vi "Read Hardware Interface Configuration.vi"(8 "error in (no error)":errorcluster, 10 "hardware interface index":u16, 11 "PLBB in":refnum<class "PL BlackBox Modbus Client.lvclass">) -> (0 "error out":errorcluster, 2 "hardware interface configuration":T1 {"UART"."flow control" items=["none", "rts", "cts", "rts/cts"]; "UART"."stop bits" items=["1", "1.5", "2"]; "UART"."parity" items=["none", "even", "odd"]}, 3 "PLBB out":refnum<class "PL BlackBox Modbus Client.lvclass">)   [LabVIEW 2015, in "PL BlackBox Modbus Client.lvclass"]
doc: "Reads the hardware interface configuration."
uses:
  PL BlackBox Modbus Client.lvclass
  <vilib>/plasmapper/PL Modbus Client/PL Modbus Client.lvclass
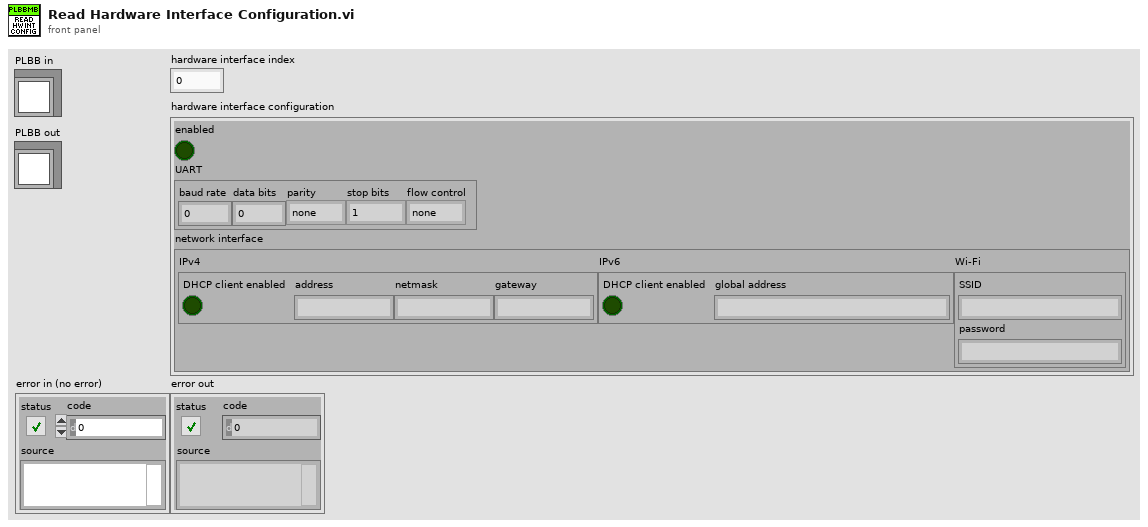
[diagram p1: front panel]
types:
  T1 = cluster{"enabled":bool, "UART":cluster{"baud rate":u32, "data bits":u16, "parity":u16, "stop bits":u16, "flow control":u16}, "network interface":cluster{"IPv4":cluster{"DHCP client enabled":bool, "address":string, "netmask":string, "gateway":string}, "IPv6":cluster{"DHCP client enabled":bool, "global address":string}, "Wi-Fi":cluster{"SSID":string, "password":string}}}
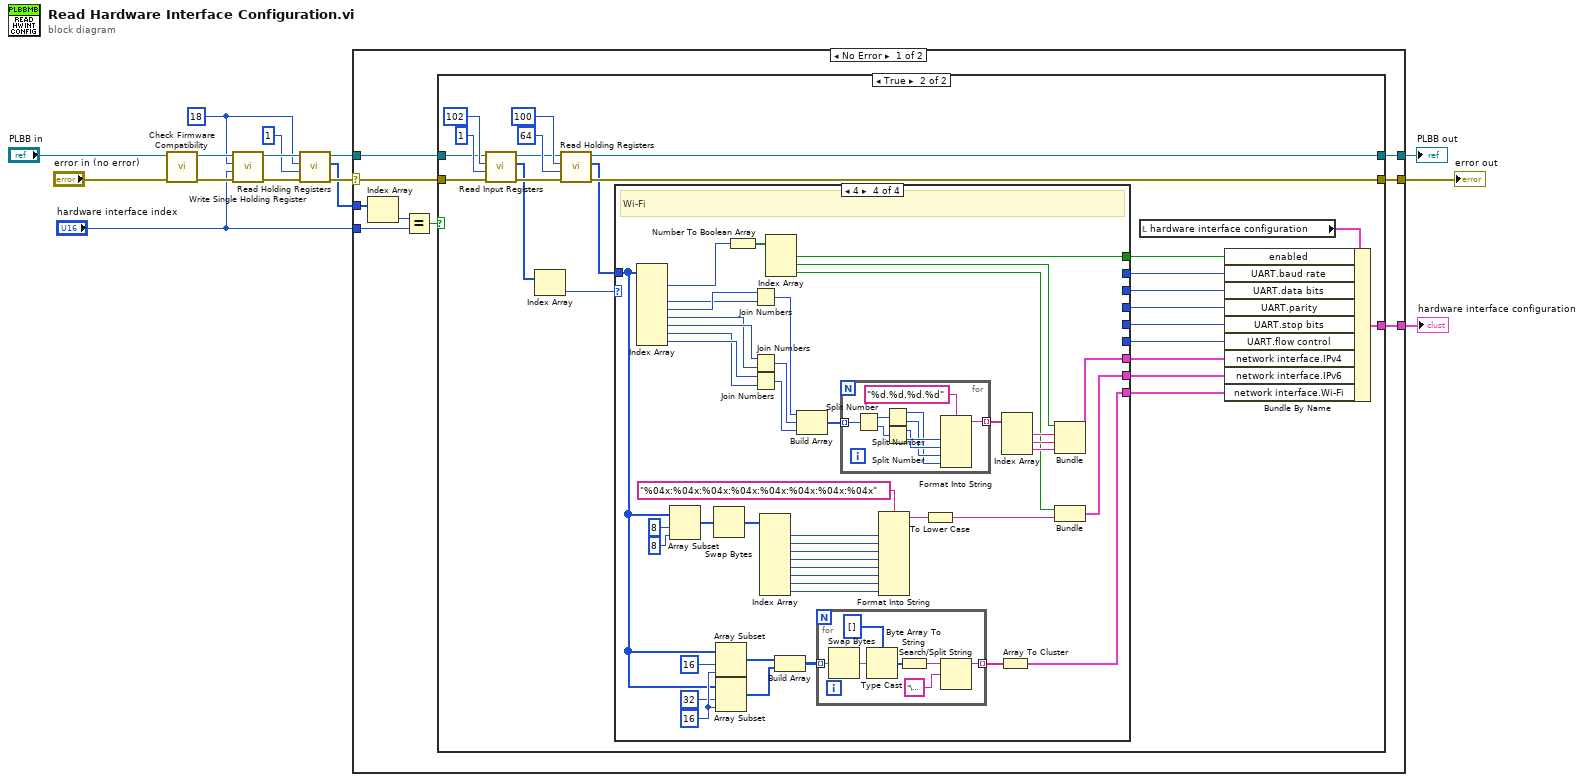
[diagram p0: block diagram]
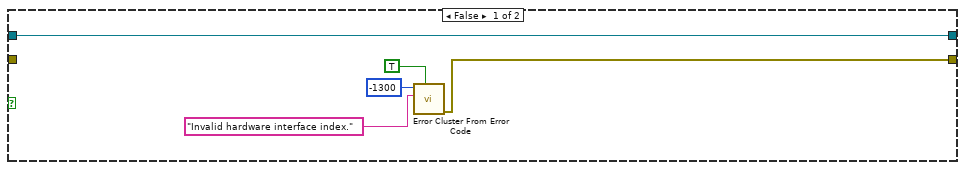
[diagram p2: hidden frame]
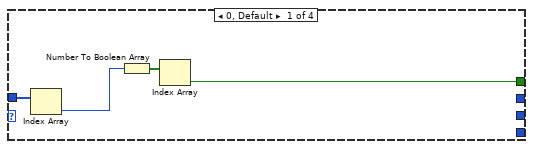
[diagram p3: hidden frame]
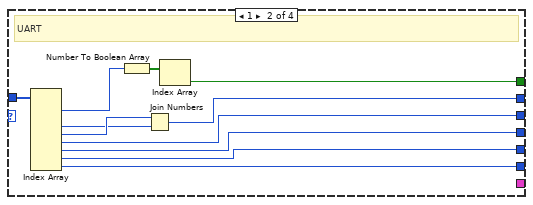
[diagram p4: hidden frame]
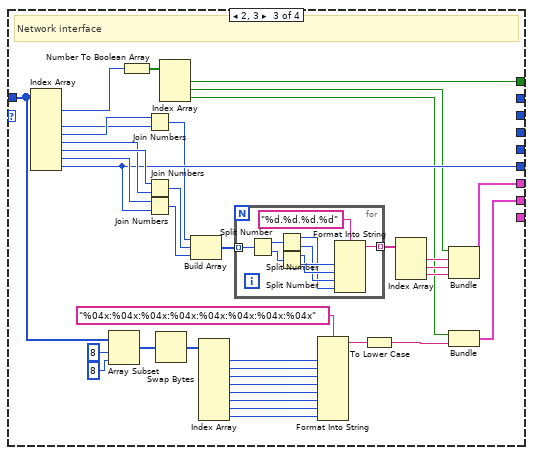
[diagram p5: hidden frame]
diagram:
  w7 = u16 18 ("address")
  n1 = call-dynamic "Check Firmware Compatibility.vi"("error in (no error)"="error in (no error)", "PLBB in"="PLBB in") -> ("error out"=w10:errorcluster, "PLBB out"=w11:refnum<class "PL BlackBox Modbus Client.lvclass">)  [unwired: 8 in]
  n2 = call <vilib>:"Write Single Holding Register.vi"("error in (no error)"=w10, "value"="hardware interface index", "address"=w7, "MODBUS in"=w11) -> ("error out"=w6:errorcluster, "MODBUS out"=w9:refnum<class "PL BlackBox Modbus Client.lvclass">)  [unwired: 6 in]
  n3 = call <vilib>:"Read Holding Registers.vi"("error in (no error)"=w6, "number of holding registers"=u16 1 ("address"), "address"=w7, "MODBUS in"=w9) -> ("error out"=w5:errorcluster, "values"=w3:u16[], "MODBUS out"=w4:refnum<class "PL BlackBox Modbus Client.lvclass">)  [unwired: 5 in]
  n4 = case shown="No Error" w5 {
    selector: w5 -> [w17 w176]
    tunnel: [w24 w176] -> w15
    tunnel: [w23 w177] -> w14
    tunnel: w4 -> [w18 w177]
    tunnel: w3 -> [w22 _]
    tunnel: "hardware interface index" -> [w20 _]
    tunnel: [w16 _] -> w1
    frame No Error {
      n5 = Index Array(array=w22) -> (element=w21:u16)  [unwired: 1 in]
      n6 = Equal?(x=w21, y=w20) -> (x = y?=w19:bool)
      n7 = case shown="True" w19 {
        tunnel: [w25 w53] -> w24
        tunnel: [w29 w52] -> w23
        tunnel: w18 -> [w29 w38]
        tunnel: w17 -> [_ w37]
        tunnel: [_ w48] -> w16
        frame False {
          n8 = call <vilib>:"Error Cluster From Error Code.vi"("show call chain? (False)"=TRUE, "error message (\"\")"="Invalid hardware interface index." ("error message (\"\")"), "error code (0)"=-1300) -> ("error out"=w25:errorcluster)  [unwired: 6 in]
        }
        frame True {
          n9 = call <vilib>:"Read Input Registers.vi"("error in (no error)"=w37, "number of input registers"=u16 1 ("address"), "address"=u16 102, "MODBUS in"=w38) -> ("error out"=w36:errorcluster, "values"=w34:u16[], "MODBUS out"=w35:refnum<class "PL BlackBox Modbus Client.lvclass">)  [unwired: 5 in]
          n10 = Index Array(array=w34) -> (element=w33:u16)  [unwired: 1 in]
          n11 = call <vilib>:"Read Holding Registers.vi"("error in (no error)"=w36, "number of holding registers"=u16 64 ("address"), "address"=u16 100, "MODBUS in"=w35) -> ("error out"=w53:errorcluster, "values"=w41:u16[], "MODBUS out"=w52:refnum<class "PL BlackBox Modbus Client.lvclass">)  [unwired: 5 in]
          n12 = case shown="4" w33 {
            tunnel: [w55 w66 w103 w157] -> w47
            tunnel: [_ w63 _ _] -> w46
            tunnel: [_ w62 _ _] -> w45
            tunnel: [_ w61 _ _] -> w44
            tunnel: [_ w60 w97 _] -> w43
            tunnel: [_ w59 _ _] -> w42
            tunnel: w41 -> [w54 w58 w78 w129]
            tunnel: [_ _ w87 w136] -> w32
            tunnel: [_ _ w85 w133] -> w31
            tunnel: [_ _ _ w131] -> w30
            frame 0, Default {
              n13 = Index Array(array=w54) -> (element=w57:u16)  [unwired: 1 in]
              n14 = Number To Boolean Array(number=w57) -> (Boolean array=w56:bool[])
              n15 = Index Array(array=w56) -> (element=w55:bool)  [unwired: 1 in]
            }
            frame 1 {
              # "UART"
              n16 = Index Array(array=w58) -> (element #1=w68:u16, element #3=w64:u16, element #4=w65:u16, element #5=w62:u16, element #6=w63:u16, element #7=w61:u16, element #8=w60:u16)  [unwired: 8 in, 1 out]
              n17 = Number To Boolean Array(number=w68) -> (Boolean array=w67:bool[])
              n18 = Join Numbers(hi=w65, lo=w64) -> ((hi.lo)=w59:u32)
              n19 = Index Array(array=w67) -> (element=w66:bool)  [unwired: 1 in]
            }
            frame 2, 3 {
              # "Network interface"
              n20 = Index Array(array=w78) -> (element #1=w105:u16, element #3=w101:u16, element #4=w102:u16, element #5=w99:u16, element #6=w100:u16, element #7=w98:u16, element #8=w97:u16)  [unwired: 8 in, 1 out]
              n21 = Array Subset(array=w78, index=8, length=8) -> (w82:u16[])
              n22 = Number To Boolean Array(number=w105) -> (Boolean array=w104:bool[])
              n23 = Join Numbers(hi=w102, lo=w101) -> ((hi.lo)=w96:u32)
              n24 = Join Numbers(hi=w100, lo=w99) -> ((hi.lo)=w95:u32)
              n25 = Join Numbers(hi=w98, lo=w97) -> ((hi.lo)=w94:u32)
              n26 = Swap Bytes(anything=w82) -> (byte swapped=w69:u16[])
              n27 = Index Array(array=w104) -> (element #1=w103:bool, element #2=w88:bool, element #3=w86:bool)  [unwired: 3 in]
              n28 = Build Array(w96, w95, w94) -> (w93:u32[])
              n29 = Index Array(array=w69) -> (element #1=w77:u16, element #2=w76:u16, element #3=w75:u16, element #4=w74:u16, element #5=w73:u16, element #6=w72:u16, element #7=w71:u16, element #8=w70:u16)  [unwired: 8 in]
              n30 = for {
                tunnel: w93 -> [w114] mode=indexing
                tunnel: [w106] -> w92 mode=indexing
                n31 = Split Number(x=w114) -> (hi(x)=w113:u16, lo(x)=w112:u16)
                n32 = Split Number(x=w113) -> (hi(x)=w107:u8, lo(x)=w108:u8)
                n33 = Split Number(x=w112) -> (hi(x)=w109:u8, lo(x)=w110:u8)
                n34 = Format Into String(format string="%d.%d.%d.%d", w110, w109, w108, w107) -> (resulting string=w106:string)  [unwired: 2 in, 1 out]
              }
              n35 = Format Into String(format string="%04x:%04x:%04x:%04x:%04x:%04x:%04x:%04x", w77, w76, w75, w74, w73, w72, w71, w70) -> (resulting string=w83:string)  [unwired: 2 in, 1 out]
              n36 = To Lower Case(string=w83) -> (all lower case string=w79:string)
              n37 = Index Array(array=w92) -> (element #1=w91:string, element #2=w89:string, element #3=w90:string)  [unwired: 3 in]
              n38 = Bundle(w88, w91, w89, w90) -> (w87:cluster{bool, string, string, string})  [unwired: 1 in]
              n39 = Bundle(w86, w79) -> (w85:cluster{bool, string})  [unwired: 1 in]
            }
            frame 4 {
              w143 = 16 ("index")
              # "Wi-Fi"
              n40 = Index Array(array=w129) -> (element #1=w159:u16, element #3=w155:u16, element #4=w156:u16, element #5=w153:u16, element #6=w154:u16, element #7=w115:u16, element #8=w116:u16)  [unwired: 8 in, 1 out]
              n41 = Array Subset(array=w129, index=8, length=8) -> (w128:u16[])
              n42 = Swap Bytes(anything=w128) -> (byte swapped=w117:u16[])
              n43 = Array Subset(array=w129, index=16, length=w143) -> (w144:u16[])
              n44 = Array Subset(array=w129, index=32, length=w143) -> (w145:u16[])
              n45 = Number To Boolean Array(number=w159) -> (Boolean array=w158:bool[])
              n46 = Join Numbers(hi=w156, lo=w155) -> ((hi.lo)=w152:u32)
              n47 = Join Numbers(hi=w154, lo=w153) -> ((hi.lo)=w151:u32)
              n48 = Join Numbers(hi=w116, lo=w115) -> ((hi.lo)=w150:u32)
              n49 = Index Array(array=w117) -> (element #1=w125:u16, element #2=w124:u16, element #3=w123:u16, element #4=w122:u16, element #5=w121:u16, element #6=w120:u16, element #7=w119:u16, element #8=w118:u16)  [unwired: 8 in]
              n50 = Index Array(array=w158) -> (element #1=w157:bool, element #2=w137:bool, element #3=w134:bool)  [unwired: 3 in]
              n51 = Build Array(w144, w145) -> (w146:u16[][])
              n52 = Build Array(w152, w151, w150) -> (w149:u32[])
              n53 = for {
                tunnel: [w161] -> w132 mode=indexing
                tunnel: w146 -> [w160] mode=indexing
                n54 = Swap Bytes(anything=w160) -> (byte swapped=w164:u16[])
                n55 = Type Cast(type=u8[] [] ("values"), x=w164) -> (*(type *) &x=w166:u8[])
                n56 = Byte Array To String(unsigned byte array=w166) -> (string=w163:string)
                n57 = Search/Split String(string=w163, search string/char (-)="\u0000") -> (substring before match=w161:string)  [unwired: 1 in, 2 out]
              }
              n58 = for {
                tunnel: w149 -> [w175] mode=indexing
                tunnel: [w167] -> w148 mode=indexing
                n59 = Split Number(x=w175) -> (hi(x)=w174:u16, lo(x)=w173:u16)
                n60 = Split Number(x=w174) -> (hi(x)=w168:u8, lo(x)=w169:u8)
                n61 = Split Number(x=w173) -> (hi(x)=w170:u8, lo(x)=w171:u8)
                n62 = Format Into String(format string="%d.%d.%d.%d", w171, w170, w169, w168) -> (resulting string=w167:string)  [unwired: 2 in, 1 out]
              }
              n63 = Format Into String(format string="%04x:%04x:%04x:%04x:%04x:%04x:%04x:%04x", w125, w124, w123, w122, w121, w120, w119, w118) -> (resulting string=w135:string)  [unwired: 2 in, 1 out]
              n64 = To Lower Case(string=w135) -> (all lower case string=w130:string)
              n65 = Array To Cluster(array=w132) -> (cluster=w131:cluster{"[0]":string, "[1]":string})
              n66 = Index Array(array=w148) -> (element #1=w140:string, element #2=w138:string, element #3=w139:string)  [unwired: 3 in]
              n67 = Bundle(w137, w140, w138, w139) -> (w136:cluster{bool, string, string, string})  [unwired: 1 in]
              n68 = Bundle(w134, w130) -> (w133:cluster{bool, string})  [unwired: 1 in]
            }
          }
          n69 = local read "hardware interface configuration"() -> (w49:T1)
          n70 = Bundle By Name(cluster=w49, "enabled"=w47, "UART.baud rate"=w42, "UART.data bits"=w45, "UART.parity"=w46, "UART.stop bits"=w44, "UART.flow control"=w43, "network interface.IPv4"=w32, "network interface.IPv6"=w31, "network interface.Wi-Fi"=w30) -> (w48:T1)
        }
      }
    }
    frame Error {
    }
  }
  "error out" <- w15
  "PLBB out" <- w14
  "hardware interface configuration" <- w1
